vi "Clear Metadata.vi"(8 "error in (no error)":errorcluster, 11 "Macro in":refnum<class "Macro.lvclass">) -> (0 "error out":errorcluster, 3 "Macro out":refnum<class "Macro.lvclass">)   [LabVIEW 2020, in "MacroAssert.lvlib" / "Macro.lvclass"]
doc: "Clears <B>Macro</B> in preparation to create a new macro with some starting information."
uses:
  Macro.lvclass
  Macro.lvclass/Macro.ctl
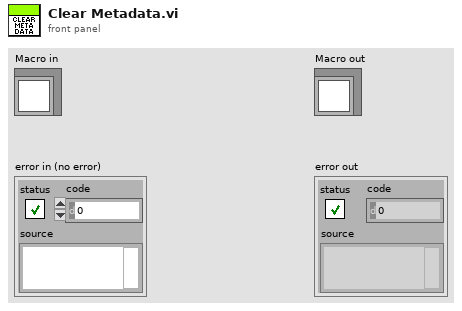
[diagram p1: front panel]
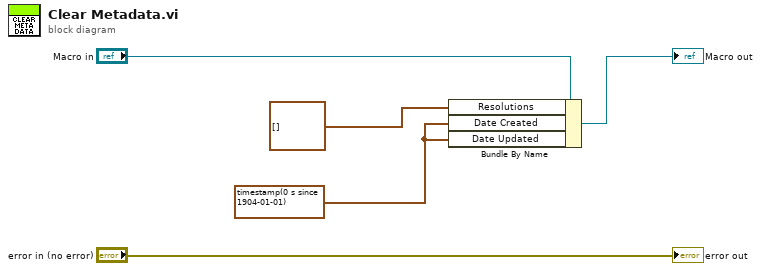
[diagram p0: block diagram]
diagram:
  w2 = timestamp(0 s since 1904-01-01) ("Date Created")
  n1 = Bundle By Name(cluster="Macro in", "Resolutions"=cluster{"Width":i16, "Height":i16}[] [], "Date Created"=w2, "Date Updated"=w2) -> (→"Macro out":refnum<class "Macro.lvclass">)
  "error out" <- "error in (no error)"
